vi "Update Analog Multiple.vi"(8 "error in (no error)":errorcluster, 10 "Channels":T1[](array[typedef]), 11 "SoftVar Module in":refnum<class "SoftVar Module.lvclass">) -> (0 "error out":errorcluster, 3 "SoftVar Module out":refnum<class "SoftVar Module.lvclass">)   [LabVIEW 2020, in "Volatus.lvlib" / "SoftVar Module.lvclass"]
uses:
  SoftVar Module.lvclass
  SoftVar Module.lvclass/SoftVar Module.ctl
  Batch Update.ctl
  <vilib>/Utility/miscctls.llb/LVMapReplaceAction.ctl
  lv-vecto/Vecto/Group/Group.lvclass
  VolatusAPI/VolatusAPI.lvclass
  Module/Module.lvclass
  C:/dev/lv20CE/relink/lv-volatus/Volatus/Module/Module.lvclass
  C:/dev/lv20CE/relink/lv-volatus/Volatus/SoftVar Module/SoftVar Module.lvclass
  messages/CmdAnalog/Data.ctl
  messages/CmdAnalog/CmdAnalog.lvlib
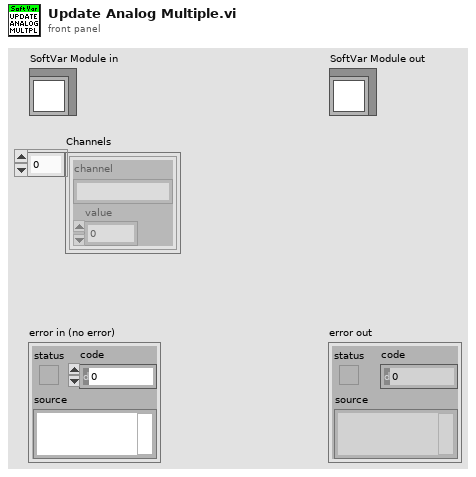
[diagram p1: front panel]
types:
  T1 = typedef "CmdAnalog.lvlib/Data.ctl" = cluster{"channel":string, "value":dbl}
  T2 = typedef "LVMapReplaceAction.ctl" = enum32{"Modify Entry only if found", "Add or Modify Entry", "Delete Entry"}
  T3 = typedef "Volatus.lvlib/SoftVar Module.lvclass/Batch Update.ctl" = cluster{"Indices":i32[], "Values":dbl[]}
  T4 = typedef "Volatus.lvlib/SoftVar Module.lvclass/Channel Info.ctl" = cluster{"Group Name":string, "Group Index":i32, "Index":i32}
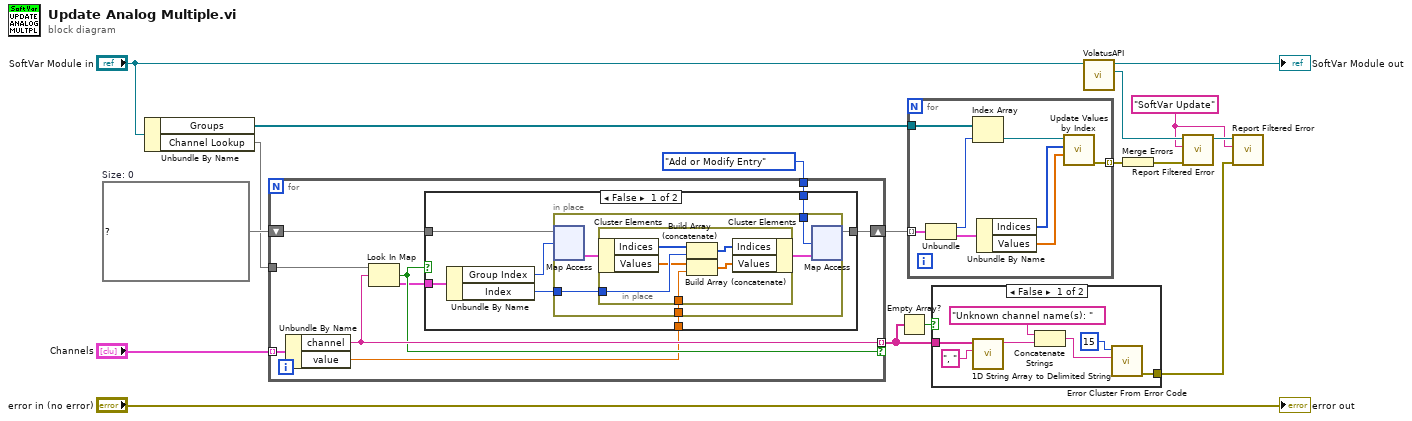
[diagram p0: block diagram]
diagram:
  w2 = "SoftVar Update" ("Context")
  w15 = map{i32, T3} {}  # Size: 0
  n1 = Unbundle By Name("SoftVar Module in") -> ("Groups"=w11:refnum<class "Group.lvclass">[], "Channel Lookup"=w14:map{string, T4})
  n2 = for {
    tunnel: "Channels" -> [w26] mode=indexing
    shift-right: [w20] -> w12
    shift-left: w15 -> [w21]
    tunnel: w14 -> [w25]
    tunnel: [w24] -> w8 mode=indexing if=w23
    tunnel: LVMapReplaceAction."Add or Modify Entry" ("action") -> [w18]
    n3 = Unbundle By Name(w26) -> ("channel"=w24:string, "value"=w19:dbl)
    n4 = Look In Map(map=w25, key=w24) -> (key not found?=w23:bool, value=w22:T4)  [unwired: 1 in]
    n5 = case shown="False" w23 {
      tunnel: w22 -> [w33 _]
      tunnel: w21 -> [w32 w45]
      tunnel: [w28 w45] -> w20
      tunnel: w19 -> [w29 _]
      tunnel: w18 -> [w27 _]
      frame False {
        n6 = Unbundle By Name(w33) -> ("Group Index"=w31:i32, "Index"=w30:i32)
        n7 = in-place {
          in-place-border: w30 -> [w37]
          in-place-border: w29 -> [w36]
          in-place-border: w27 -> [w34]
          n8 = in-place-map #1(w32, w31) -> (w38:T3)  [unwired: 1 in, 1 out]
          n9 = in-place {
            in-place-border: w37 -> [w43]
            in-place-border: w36 -> [w39]
            n10 = in-place-cluster #2(w38) -> ("Indices"=w44:i32[], "Values"=w42:dbl[])
            n11 = Build Array (concatenate)(w44, w43) -> (w40:i32[])
            n12 = Build Array (concatenate)(w42, w39) -> (w41:dbl[])
            n13 = in-place-cluster #2("Indices"=w40, "Values"=w41) -> (w35:T3)
          }
          n14 = in-place-map #1(w35, w34) -> (w28:map{i32, T3})  [unwired: 2 out]
        }
      }
      frame True {
      }
    }
  }
  n15 = Empty Array?(array=w8) -> (empty?=w9:bool)
  n16 = for {
    tunnel: w12 -> [w53] mode=indexing
    tunnel: w11 -> [w52]
    tunnel: [w46] -> w10 mode=indexing
    n17 = Unbundle(w53) -> ("Group Index"=w51:i32, "Batch Update"=w50:T3)
    n18 = Index Array(array=w52, index=w51) -> (element=w49:refnum<class "Group.lvclass">)
    n19 = Unbundle By Name(w50) -> ("Indices"=w48:i32[], "Values"=w47:dbl[])
    n20 = call "Update Values by Index.vi"("Scaled"=w47, "Index"=w48, "Group in"=w49) -> ("error out"=w46:errorcluster)  [unwired: 7 in, 1 out]
  }
  n21 = case shown="False" w9 {
    tunnel: w8 -> [w60 _]
    tunnel: [w54 _] -> w1
    frame False {
      n22 = call <vilib>:"1D String Array to Delimited String.vi"("delimiter"=", ", "string array"=w60) -> ("delimited string"=w57:string)  [unwired: 9 in]
      n23 = Concatenate Strings("Unknown channel name(s): ", w57) -> (w55:string)
      n24 = call <vilib>:"Error Cluster From Error Code.vi"("error message (\"\")"=w55, "error code (0)"=15) -> ("error out"=w54:errorcluster)  [unwired: 7 in]
    }
    frame True {
    }
  }
  n25 = call "VolatusAPI.vi"("Module in"="SoftVar Module in") -> ("VolatusAPI"=w4:refnum<class "VolatusAPI.lvclass">, "Module out"=→"SoftVar Module out":refnum<class "SoftVar Module.lvclass">)  [unwired: 9 in]
  n26 = Merge Errors(w10) -> (w7:errorcluster)
  n27 = call "Report Filtered Error.vi"("error in (no error)"=w7, "Context"=w2, "VolatusAPI in"=w4) -> ("VolatusAPI out"=w3:refnum<class "VolatusAPI.lvclass">)  [unwired: 7 in, 1 out]
  n28 = call "Report Filtered Error.vi"("error in (no error)"=w1, "Context"=w2, "VolatusAPI in"=w3) -> ()  [unwired: 7 in, 2 out]
  "error out" <- "error in (no error)"
